vi "SR Bistable.vi"(8 "error in":errorcluster, 10 "reset":bool, 11 "set":bool) -> (0 "error out":errorcluster, 3 "output":bool)   [LabVIEW 2020, in "NI_FunctionBlock Libraries.lvlib"]
uses:
  <vilib>/functionblocks/NI_FunctionBlock Libraries.lvlib
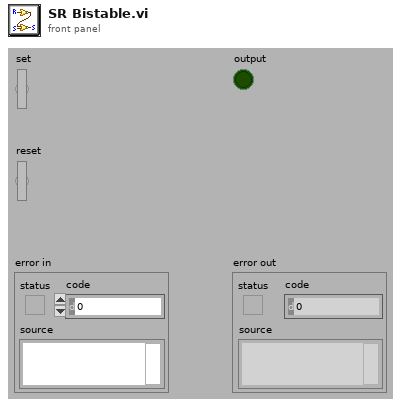
[diagram p1: front panel]
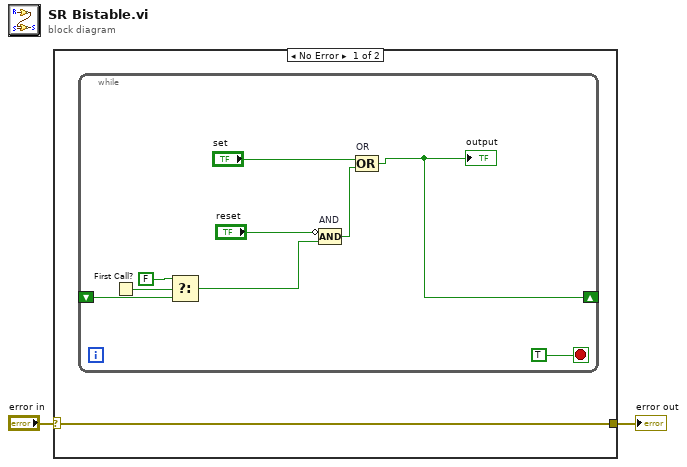
[diagram p0: block diagram]
diagram:
  n1 = case shown="No Error" "error in" {
    selector: "error in" -> [w3 w13]
    tunnel: [w3 w13] -> w1
    frame No Error {
      n2 = while {
        shift-right: [w5] -> _
        shift-left: _ -> [w6]
        stop <- TRUE stop-if-true
        n3 = First Call?() -> (First Call?: T/F=w10:bool)
        n4 = Select(t=FALSE, s=w10, f=w6) -> (s? t:f=w8:bool)
        n5 = Compound Arithmetic op=AND "AND"(invert "reset", w8) -> (w7:bool)
        n6 = Compound Arithmetic op=OR "OR"("set", w7) -> (w5:bool)
        "output" <- w5
      }
    }
    frame Error {
    }
  }
  "error out" <- w1
